vi "solar - pwm and displaz.vi"() -> ()   [LabVIEW 2020]
uses:
  <vilib>/MakerHub/LINX/Public/Peripherals/Analog/Analog Read 1 Chan.vi
  <vilib>/MakerHub/LINX/Public/Peripherals/PWM/PWM Set Duty Cycle 1 Chan.vi
  <vilib>/MakerHub/LINX/Public/Peripherals/Analog/Analog Read N Chans.vi
  <vilib>/MakerHub/LINX/Private/Local IO/LinxAnalogRead.vi
  <vilib>/MakerHub/LINX/Public/Utilities/Check Channel.vi
  <vilib>/MakerHub/LINX/Public/Utilities/Open Serial.vi
  <vilib>/MakerHub/LINX/Private/Utilties/Generate Error.vi
  <vilib>/MakerHub/LINX/Public/Peripherals/PWM/PWM Set Duty Cycle N Chans.vi
  <vilib>/MakerHub/LINX/LMH-LINX.lvlib
panel:
  out "x/y":dbl
  out "sum":dbl
  out "Waveform Chart":dbl(graph)
  out "Error Out 2":errorcluster
  out "Error Out":errorcluster
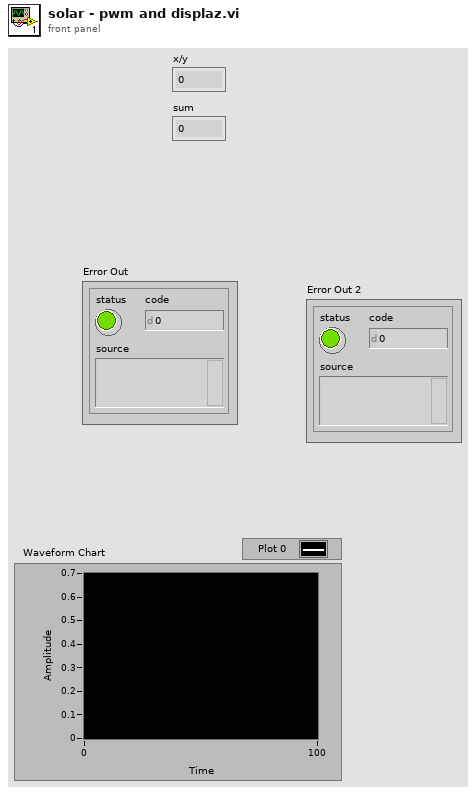
[diagram p1: front panel]
types:
  T1 = typedef "LMH-LINX.lvlib/LINX Ref.ctl" = cluster{"IO":T2, "Interface":T3, "LINX Device Config":T4}
  T2 = typedef "LMH-LINX.lvlib/Platform.ctl" = enum16{"Remote", "Local"}
  T3 = typedef "LMH-LINX.lvlib/Interface.ctl" = enum16{"Serial", "TCP"}
  T4 = typedef "LMH-LINX.lvlib/Device.lvlib/LINX Device Config.ctl" = cluster{"Interface":T3, "COM Port":refnum<visa-resource-name>, "TCP Configuration":T5, "Device Family":u8, "Device ID":u8, "Device Name":string, "TCP Ref":refnum<k5>, "Channels":T6}
  T5 = typedef "LMH-LINX.lvlib/Device.lvlib/TCP Config.ctl" = cluster{"IP Address":string, "Port":u16}
  T6 = typedef "LMH-LINX.lvlib/Channels.ctl" = cluster{"DI":u8[], "DO":u8[], "AI":u8[], "AO":u8[], "PWM":u8[], "QE":u8[], "UART":u8[], "I2C 2":u8[], "SPI":u8[], "CAN":u8[], "Servo":u8[], "AI Ref (V)":dbl, "AI Resolution (Bits)":u8, "AO Ref (V)":dbl, "AO Resolution (Bits)":u8}
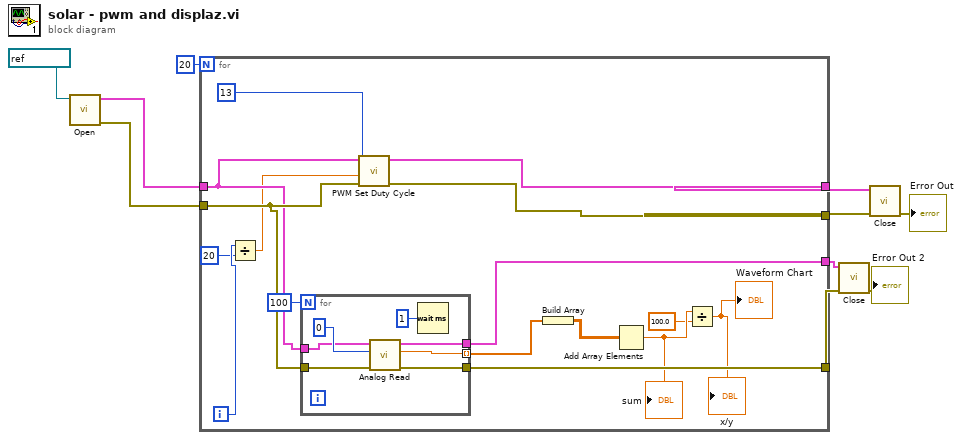
[diagram p0: block diagram]
diagram:
  n1 = call-poly <vilib>:"Open.vi"("Serial Port"=refnum<visa-resource-name> "COM4") -> ("Error Out"=w3:errorcluster, "LINX Resource"=w6:T1)  [unwired: 8 in, 1 out]
  n2 = for {
    N: 20 -> [_]
    tunnel: [w22] -> w7
    tunnel: w6 -> [w21]
    tunnel: [w25] -> w5
    tunnel: [w24] -> w4
    tunnel: w3 -> [w23]
    tunnel: [w20] -> w2
    i -> [w15]
    n3 = Divide(x=w15, y=20) -> (x/y=w13:dbl)
    n4 = for {
      N: 100 -> [_]
      tunnel: w23 -> [w32]
      tunnel: [w31] -> w22
      tunnel: w21 -> [w30]
      tunnel: [w29] -> w20
      tunnel: [w28] -> w19 mode=indexing
      n5 = call-poly <vilib>:"Analog Read.vi"("Error In"=w32, "Analog Channel"=u8 0, "LINX Resource"=w30) -> ("Error Out"=w29:errorcluster, "Voltage"=w28:dbl, "LINX Resource"=w31:T1)  [unwired: 5 in, 1 out]
      n6 = Wait (ms)(milliseconds to wait=u32 1) -> ()  [unwired: 1 out]
    }
    n7 = call-poly <vilib>:"PWM Set Duty Cycle.vi"("Error In"=w23, "Duty Cycle (0-1)"=w13, "PWM Channel"=u8 13, "LINX Resource"=w21) -> ("Error Out"=w24:errorcluster, "LINX Resource"=w25:T1)  [unwired: 6 in]
    n8 = Build Array(w19) -> (w17:dbl[][])
    n9 = Add Array Elements(numeric array=w17) -> (sum=w16:dbl)
    "sum" <- w16
    n10 = Divide(x=w16, y=100.0) -> (x/y=→"Waveform Chart" →"x/y":dbl)
  }
  n11 = call <vilib>:"Close.vi"("Error In"=w2, "LINX Resource"=w7) -> ("Error Out"=→"Error Out 2":errorcluster)  [unwired: 9 in]
  n12 = call <vilib>:"Close.vi"("Error In"=w4, "LINX Resource"=w5) -> ("Error Out"=→"Error Out":errorcluster)  [unwired: 9 in]
